vi "Pfeiffer-RVC300.contents.vi"   [LabVIEW 2014, in "Pfeiffer-RVC300.lvlib"]
uses:
  Pfeiffer-RVC300.lvlib
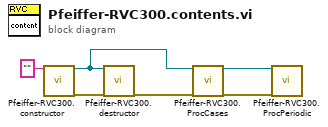
[diagram p0: block diagram]
diagram:
  n1 = call "Pfeiffer-RVC300.constructor.vi"("name"="") -> ("i ref out"=w3:refnum<vi>, "error out"=w5:errorcluster)  [unwired: 16 in, 1 out]
  n2 = call "Pfeiffer-RVC300.destructor.vi"("i ref in"=w3, "error in(no error)"=w5) -> ("error out"=w4:errorcluster)  [unwired: 17 in]
  n3 = call "Pfeiffer-RVC300.ProcCases.vi"("i ref in"=w3, "error in (no error)"=w4) -> ("i ref out"=w1:refnum<vi>, "error out"=w2:errorcluster)  [unwired: 15 in, 1 out]
  n4 = call "Pfeiffer-RVC300.ProcPeriodic.vi"("i ref in"=w1, "error in (no error)"=w2) -> ()  [unwired: 15 in, 3 out]
